vi "sub_gpsdeg_to_xydeg.vi"(11 "Heading":dbl) -> (3 "deg":dbl)   [LabVIEW 2019]
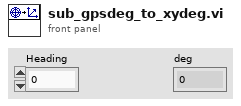
[diagram p1: front panel]
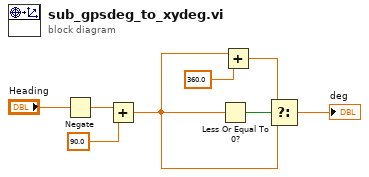
[diagram p0: block diagram]
diagram:
  n1 = Negate(x="Heading") -> (-x=w6:dbl)
  n2 = Add(x=w6, y=90.0) -> (x+y=w3:dbl)
  n3 = Less Or Equal To 0?(x=w3) -> (x <= 0?=w5:bool)
  n4 = Add(x=w3, y=360.0) -> (x+y=w1:dbl)
  n5 = Select(t=w1, s=w5, f=w3) -> (s? t:f=→"deg":dbl)
